vi "FilePaths.vi"(8 "error in":errorcluster) -> (0 "error out":errorcluster, 2 "paths":T1)   [LabVIEW 2013]
uses:
  Controls/FilePaths.ctl
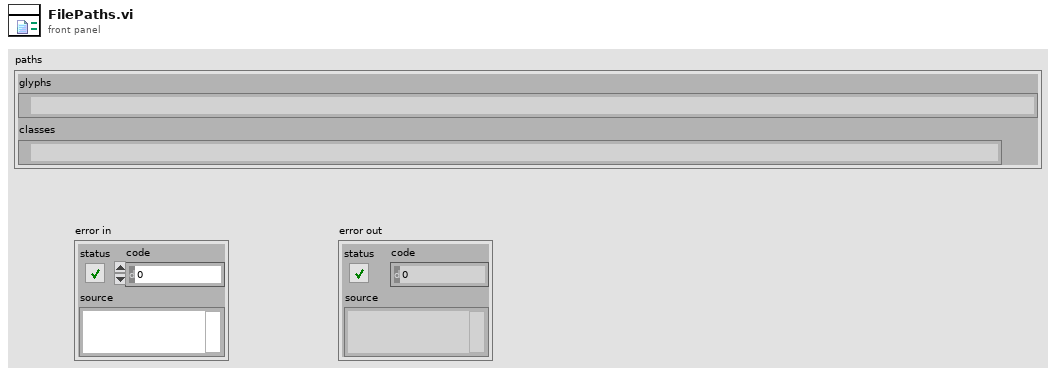
[diagram p1: front panel]
types:
  T1 = typedef "FilePaths.ctl" = cluster{"glyphs":path, "classes":path}
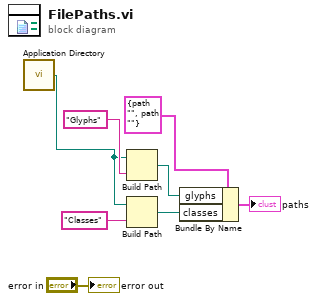
[diagram p0: block diagram]
diagram:
  n1 = call <vilib>:"Application Directory.vi"() -> ("Application Directory"=w1:path)
  n2 = Build Path(base path=w1, name or relative path="Glyphs") -> (appended path=w5:path)
  n3 = Build Path(base path=w1, name or relative path="Classes") -> (appended path=w2:path)
  n4 = Bundle By Name(cluster=T1 {"glyphs"=path "", "classes"=path ""} ("Cluster 2"), "glyphs"=w5, "classes"=w2) -> (→"paths":T1)
  "error out" <- "error in"
